vi "Parse Signed Array from String.vi"(10 "Delimiter regex":string, 11 "Input":string) -> (2 "Parsed I64 Array":i64[](array[numeric]), 3 "Parsed Array":string[](array[string]))   [LabVIEW 2020]
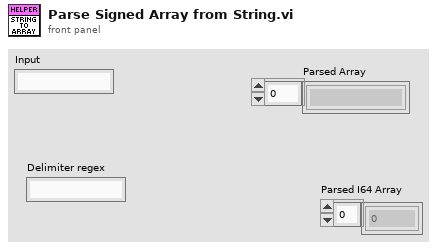
[diagram p1: front panel]
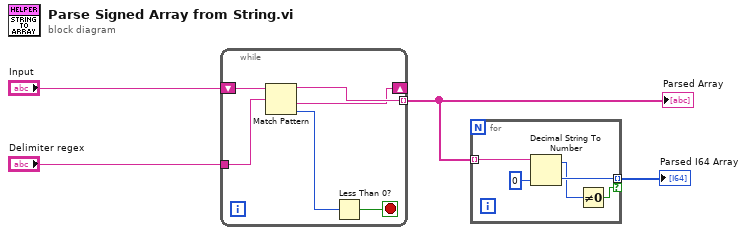
[diagram p0: block diagram]
diagram:
  n1 = while {
    tunnel: "Delimiter regex" -> [w7]
    tunnel: [w6] -> w2 mode=indexing
    shift-right: [w5] -> _
    shift-left: "Input" -> [w10]
    stop <- w9 stop-if-true
    n2 = Match Pattern(string=w10, regular expression=w7) -> (before substring=w6:string, after substring=w5:string, offset past match=w8:i32)  [unwired: 1 in, 1 out]
    n3 = Less Than 0?(x=w8) -> (x < 0?=w9:bool)
  }
  "Parsed Array" <- w2
  n4 = for {
    tunnel: w2 -> [w15] mode=indexing
    tunnel: [w13] -> w1 mode=indexing if=w11
    n5 = Decimal String To Number(string=w15, default (0L)=i64 0 ("default (0 I32)")) -> (offset past number=w12:i32, number=w13:i64)  [unwired: 1 in]
    n6 = Not Equal To 0?(x=w12) -> (x != 0?=w11:bool)
  }
  "Parsed I64 Array" <- w1
